vi "ConfigureSweep.vi"(8 "error in (no error)":errorcluster, 11 "config":T1) -> (0 "error out":errorcluster, 3 "config out":T1)   [LabVIEW 2017, in "EmsaAcquisition.lvlib"]
uses:
  <vilib>/addons/InsightCM/Devices/Shared/Emsa/EmsaAcquisition/EmsaAcquisition.lvlib
  <vilib>/addons/InsightCM/Devices/Shared/Emsa/EmsaAcquisition/controls/config.ctl
  <vilib>/addons/InsightCM/Devices/Shared/Emsa/Emsa9770API/9770 API.lvclass
  <vilib>/addons/InsightCM/Devices/Shared/Emsa/EmsaAcquisition/controls/group.ctl
  <vilib>/addons/InsightCM/Devices/Shared/Emsa/EmsaAcquisition/controls/acqConfig.ctl
  InsightCM/Devices/WebServices/Emsa/accessors/SweepStats.ctl
  <vilib>/addons/InsightCM/Utilities/DeviceModelHelpers/DeviceModelHelpers.lvlib
  <vilib>/addons/InsightCM/Utilities/GlobalConfiguration/GlobalConfiguration.lvlib
  InsightCM/Devices/WebServices/Emsa/accessors/EmsaWebServiceAccessors.lvlib
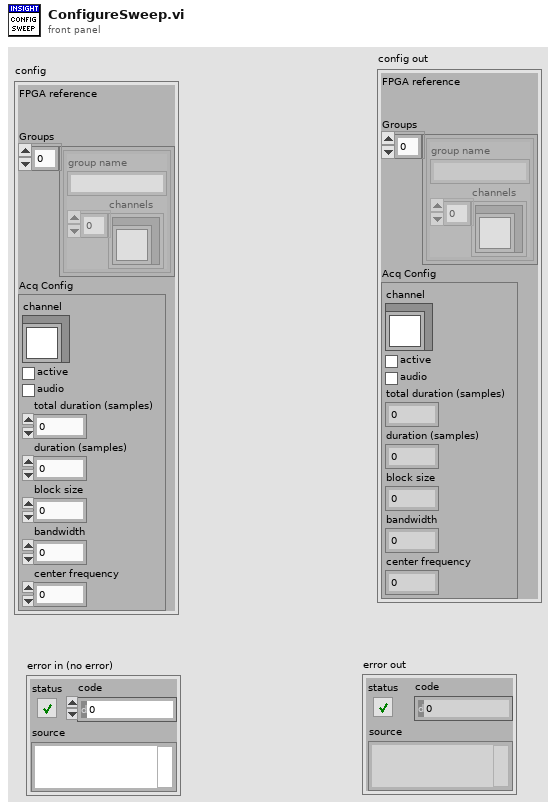
[diagram p1: front panel]
types:
  T1 = typedef "EmsaAcquisition.lvlib/config.ctl" = cluster{"FPGA reference":refnum<k20>, "Groups":T2[], "Acq Config":T3}
  T2 = typedef "EmsaAcquisition.lvlib/group.ctl" = cluster{"group name":string, "channels":refnum<class "9770 API.lvclass">[]}
  T3 = typedef "EmsaAcquisition.lvlib/acqConfig.ctl" = cluster{"channel":refnum<class "9770 API.lvclass">, "active":bool, "audio":bool, "total duration (samples)":i32, "duration (samples)":i32, "block size":i32, "bandwidth":dbl, "center frequency":dbl}
  T4 = typedef "AssetNode.ctl" = cluster{"Id":string, "Type":string, "Name":string, "ParentIds":string[], "State":T5, "MeasType":string, "Properties":T6[], "OperatingStates":T7[], "Metrics":T10[], "TrendAlarmRules":T11[], "References":T14[]}
  T5 = typedef "AssetState.ctl" = cluster{"Disabled":bool}
  T6 = typedef "KeyValuePair.ctl" = cluster{"Key":string, "Value":string}
  T7 = typedef "OperatingState.ctl" = cluster{"Name":string, "Properties":T6[], "Triggers":T8[]}
  T8 = typedef "Trigger.ctl" = cluster{"Type":string, "Expression":string, "Conditions":T9[]}
  T9 = typedef "Condition.ctl" = cluster{"Source":string, "Type":string, "Operator":string, "CompareTo":string, "DwellSeconds":dbl}
  T10 = typedef "Metric.ctl" = cluster{"Id":string, "Name":string, "Unit":string, "Properties":T6[], "MetricDefinitionInstanceId":string}
  T11 = typedef "TrendAlarmRule.ctl" = cluster{"Id":string, "AssetNodeId":string, "TrendId":string, "Disabled":bool, "OperatingState":string, "Operator":string, "Hysteresis":dbl, "OnDelaySeconds":dbl, "OffDelaySeconds":dbl, "Levels":T12[], "Properties":T6[]}
  T12 = typedef "TrendAlarmLevel.ctl" = cluster{"Severity":i32, "CompareTo":dbl, "Actions":T13[]}
  T13 = typedef "AlarmAction.ctl" = cluster{"Type":string, "Props":T6[]}
  T14 = typedef "AssetNodeReference.ctl" = cluster{"NodeId":string, "Name":string}
  T15 = typedef "R2_DeviceModel.ctl" = cluster{"Device":T16, "Channels":T20[], "Tags":T21[]}
  T16 = typedef "R2_Device.ctl" = cluster{"Id":string, "Name":string, "DeviceType":string, "HardwareName":string, "IpAddress":string, "HardwareInfo":T6[], "ApplicationType":string, "ApplicationVersion":string, "EquipmentIds":string[], "ConfigurationVersion":string, "State":T17, "Properties":T6[], "DataGroups":T18[], "BurstModeTrigger":T19}
  T17 = typedef "DeviceState.ctl" = cluster{"Disabled":bool}
  T18 = typedef "R2_DataGroup.ctl" = cluster{"Name":string, "OperatingStates":T7[], "Properties":T6[], "EquipmentIds":string[], "AssetNodeId":string}
  T19 = typedef "BurstModeTrigger.ctl" = cluster{"Trigger":T8, "SampleRate":string, "AcquisitionLength":string}
  T20 = typedef "R2_Channel.ctl" = cluster{"Id":string, "DeviceId":string, "Name":string, "ChannelType":string, "HardwareKey":string, "HardwareChannel":string, "DataGroup":string, "Keywords":string[], "EquipmentIds":string[], "Properties":T6[], "Metrics":T10[], "AssetNodeId":string, "MeasType":string, "AssetName":string}
  T21 = typedef "Tag.ctl" = cluster{"Id":string, "Path":string, "Name":string, "Datatype":string, "Props":T6[], "Keywords":string[]}
  T22 = typedef "EmsaWebServiceAccessors.lvlib/SweepStats.ctl" = cluster{"Channel":string, "Sweep Time(min)":dbl, "Current Frequency(Hz)":dbl, "Max Sweep Time(min)":dbl, "Completed Sweep":bool}
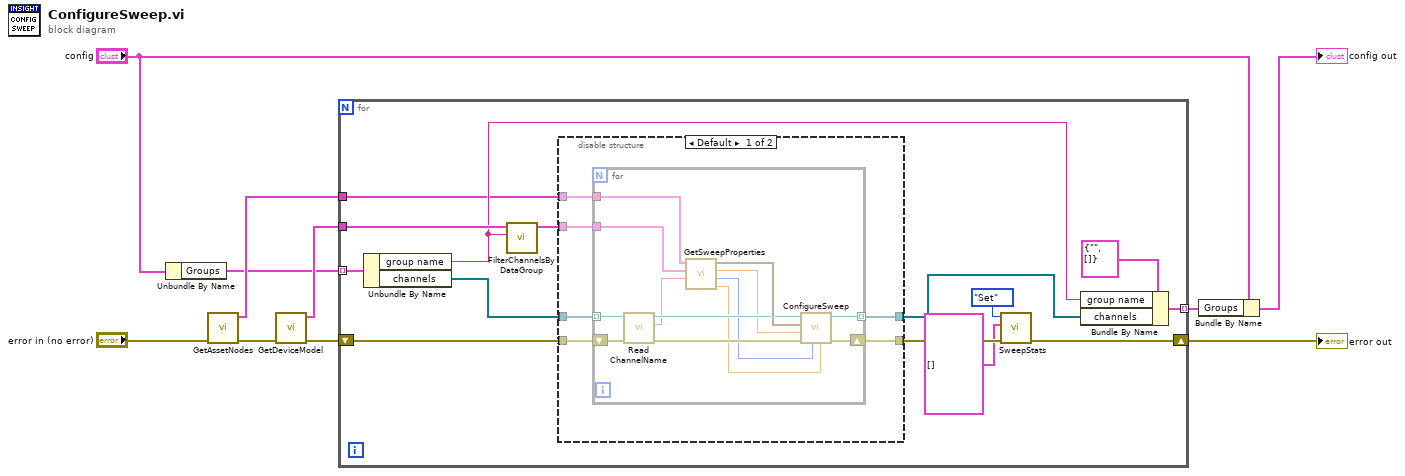
[diagram p0: block diagram]
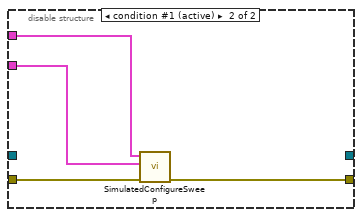
[diagram p2: hidden frame]
diagram:
  n1 = Unbundle By Name("config") -> ("Groups"=w7:T2[])
  n2 = call <vilib>:"GetAssetNodes.vi"("error in (no error)"="error in (no error)") -> ("error out"=w5:errorcluster, "AssetNodes"=w8:T4[])  [unwired: 8 in, 1 out]
  n3 = call <vilib>:"GetDeviceModel.vi"("error in (no error)"=w5) -> ("error out"=w6:errorcluster, "device model"=w10:T15)  [unwired: 8 in, 1 out]
  n4 = for {
    tunnel: w10 -> [w24]
    shift-right: [w12] -> w9
    shift-left: w6 -> [w23]
    tunnel: [w21] -> w3 mode=indexing
    tunnel: w8 -> [w18]
    tunnel: w7 -> [w17] mode=indexing
    n5 = Unbundle By Name(w17) -> ("group name"=w20:string, "channels"=w19:refnum<class "9770 API.lvclass">[])
    n6 = call <vilib>:"FilterChannelsByDataGroup.vi"("group"=w20, "device model"=w24) -> ("channels in data group"=w22:T20[])  [unwired: 8 in, 1 out]
    n7 = disable-structure shown="Default" {
      disable-tunnel: [w30 w47] -> w13
      disable-tunnel: w23 -> [w29 w46]
      disable-tunnel: w22 -> [w28 w45]
      disable-tunnel: [w27 _] -> w14
      disable-tunnel: w19 -> [w26 _]
      disable-tunnel: w18 -> [w25 w44]
      frame condition #0 {
        n8 = for {
          tunnel: w28 -> [w38]
          shift-right: [w43] -> w30
          shift-left: w29 -> [w40]
          tunnel: [w42] -> w27 mode=indexing
          tunnel: w26 -> [w41] mode=indexing
          tunnel: w25 -> [w39]
          n9 = call <vilib>:"Read ChannelName.vi"("error in (no error)"=w40, "9770 API in"=w41) -> ("error out"=w34:errorcluster, "ChannelName"=w35:string, "9770 API out"=w36:refnum<class "9770 API.lvclass">)  [unwired: 7 in]
          n10 = call <vilib>:"GetSweepProperties.vi"("channel"=w35, "data group channels"=w38, "asset nodes"=w39) -> ("full scale voltage"=w31:dbl, "DetectionMode"=w32:enum16{"Peak", "Quasi Peak", "Average"}, "detection time"=w33:dbl, "sweep freq list"=w37:cluster{"frequency":dbl, "bandwidth":dbl}[])  [unwired: 4 in, 1 out]
          n11 = call <vilib>:"ConfigureSweep.vi"("FullScaleVoltage"=w31, "DetectionMode"=w32, "error in (no error)"=w34, "DetectionTime"=w33, "Sweep"=w37, "9770 API in"=w36) -> ("error out"=w43:errorcluster, "9770 API out"=w42:refnum<class "9770 API.lvclass">)  [unwired: 4 in]
        }
      }
      frame condition #1 (active) {
        n12 = call <vilib>:"SimulatedConfigureSweep.vi"("error in (no error)"=w46, "channels in data group"=w45, "AssetNodes"=w44) -> ("error out"=w47:errorcluster)  [unwired: 8 in]
      }
    }
    n13 = call "SweepStats.vi"("error in (no error)"=w13, "Sweep Stats"=T22[] [], "Action"=enum16{"Get", "Set"}."Set") -> ("error out"=w12:errorcluster)  [unwired: 7 in, 1 out]
    n14 = Bundle By Name(cluster=T2 {"group name"="", "channels"=[]}, "group name"=w20, "channels"=w14) -> (w21:T2)
  }
  "error out" <- w9
  n15 = Bundle By Name(cluster="config", "Groups"=w3) -> (→"config out":T1)
